vi "To Serial Form.vi"(6 "Serial Version":T1, 10 "Serializer in":refnum<class "Serializer.lvclass">, 11 "cCRDS in":refnum<class "cCRDS.lvclass">) -> (0 "error out":errorcluster, 2 "Serializer out":refnum<class "Serializer.lvclass">, 3 "cCRDS out":refnum<class "cCRDS.lvclass">)   [LabVIEW 2012]
uses:
  <userlib>/Serialization/Serializable/Serializable.lvclass
  <userlib>/Serialization/Serializable/Insert Serializable.vi
  <userlib>/Serialization/Serializable/Insert Boolean.vi
  <userlib>/Serialization/Serializer/Serializer.lvclass
  <userlib>/Serialization/Serialization Common/Serial Version.ctl
  <userlib>/Serialization/Serialization Common/Serialization Common.lvlib
  cCRDS.lvclass
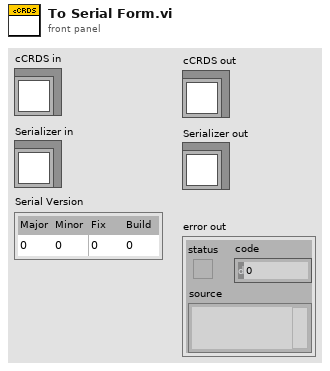
[diagram p1: front panel]
types:
  T1 = typedef "Serialization Common.lvlib/Serial Version.ctl" = cluster{"Major":u16, "Minor":u16, "Fix":u16, "Build":u16}
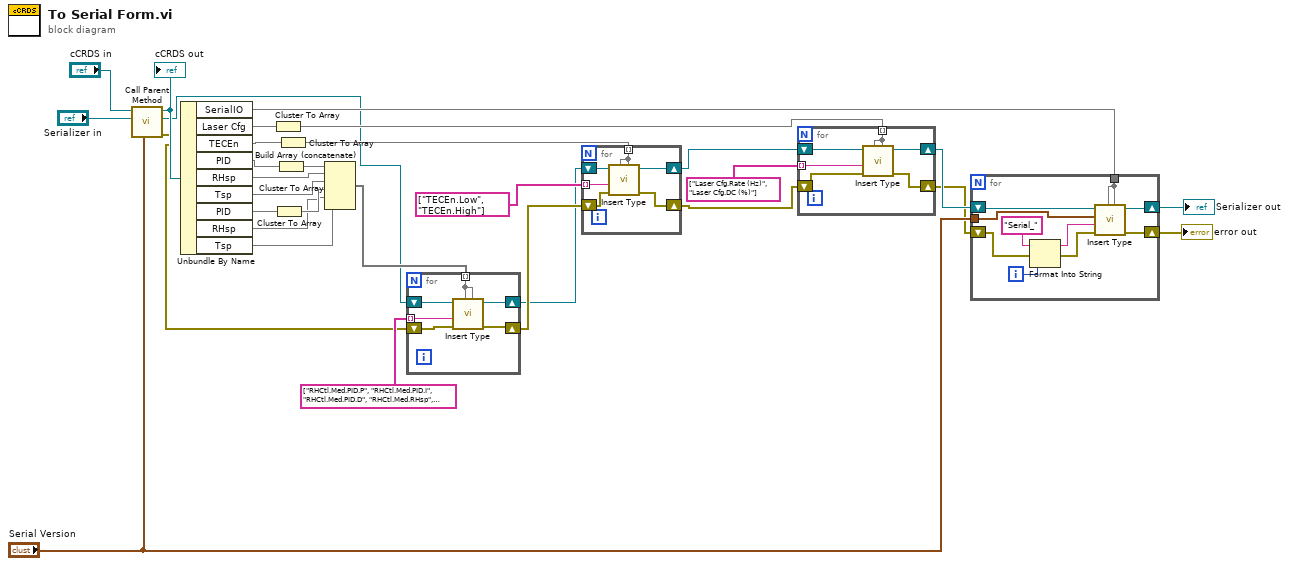
[diagram p0: block diagram]
diagram:
  n1 = call-parent "Call Parent Method"("Serial Version"="Serial Version", "Serializer in"="Serializer in", "Instrument in"="cCRDS in") -> ("error out"=w6:errorcluster, "Serializer out"=w2:refnum<class "Serializer.lvclass">, "Instrument out"=w28:refnum<class "cCRDS.lvclass">)  [unwired: 6 in]
  "cCRDS out" <- w28
  n2 = Unbundle By Name(w28) -> ("SerialIO"=w29, "Laser Cfg"=w24, "TECEn"=w21, "PID"=w16, "RHsp"=w14, "Tsp"=w13, "PID"=w12, "RHsp"=w10, "Tsp"=w9)
  n3 = Cluster To Array(cluster=w24) -> (array=w23:void[])
  n4 = Cluster To Array(cluster=w12) -> (array=w11:void[])
  n5 = Cluster To Array(cluster=w16) -> (array=w15:void[])
  n6 = Cluster To Array(cluster=w21) -> (array=w20:void[])
  n7 = Build Array (concatenate)(w15, w14, w13, w11, w10, w9) -> (w8:void[])
  n8 = for {
    tunnel: w8 -> [w37] mode=indexing
    shift-right: [w36] -> w1
    shift-left: w2 -> [w35]
    tunnel: string[] ["RHCtl.Med.PID.P", "RHCtl.Med.PID.I", "RHCtl.Med.PID.D", "RHCtl.Med.RHsp", "RHCtl.Med.Tsp", "RHCtl.High.PID.P", "RHCtl.High.PID.I", "RHCtl.High.PID.D", "RHCtl.High.RHsp", "RHCtl.High.Tsp"] -> [w34] mode=indexing
    shift-right: [w32] -> w5
    shift-left: w6 -> [w33]
    n9 = call-poly <userlib>:"Insert Type.vi"("Boolean"=w37, "Default Value"=w37, "error in (no error)"=w33, "Name"=w34, "Serializer in"=w35) -> ("error out"=w32:errorcluster, "Serializer out"=w36:refnum<class "Serializer.lvclass">)  [unwired: 5 in]
  }
  n10 = for {
    tunnel: w20 -> [w43] mode=indexing
    shift-right: [w41] -> w18
    shift-left: w1 -> [w42]
    tunnel: string[] ["TECEn.Low", "TECEn.High"] -> [w40] mode=indexing
    shift-right: [w38] -> w4
    shift-left: w5 -> [w39]
    n11 = call-poly <userlib>:"Insert Type.vi"("Boolean"=w43, "Default Value"=w43, "error in (no error)"=w39, "Name"=w40, "Serializer in"=w42) -> ("error out"=w38:errorcluster, "Serializer out"=w41:refnum<class "Serializer.lvclass">)  [unwired: 5 in]
  }
  n12 = for {
    tunnel: w23 -> [w49] mode=indexing
    shift-right: [w47] -> w17
    shift-left: w18 -> [w48]
    tunnel: string[] ["Laser Cfg.Rate (Hz)", "Laser Cfg.DC (%)"] -> [w46] mode=indexing
    shift-right: [w44] -> w3
    shift-left: w4 -> [w45]
    n13 = call-poly <userlib>:"Insert Type.vi"("Boolean"=w49, "Default Value"=w49, "error in (no error)"=w45, "Name"=w46, "Serializer in"=w48) -> ("error out"=w44:errorcluster, "Serializer out"=w47:refnum<class "Serializer.lvclass">)  [unwired: 5 in]
  }
  n14 = for {
    tunnel: w29 -> [w59]
    shift-right: [w57] -> w26
    shift-left: w17 -> [w58]
    shift-right: [w56] -> w25
    shift-left: w3 -> [w52]
    tunnel: "Serial Version" -> [w50]
    i -> [w55]
    n15 = Format Into String(initial string="Serial_", error in=w52, w55) -> (resulting string=w53:string, error out=w51:errorcluster)  [unwired: 1 in]
    n16 = call-poly <userlib>:"Insert Type.vi"("Serializable"=w59, "Default Value"=w59, "error in (no error)"=w51, "Name"=w53, "Serial Version"=w50, "Serializer in"=w58) -> ("error out"=w56:errorcluster, "Serializer out"=w57:refnum<class "Serializer.lvclass">)  [unwired: 4 in]
  }
  "error out" <- w25
  "Serializer out" <- w26
